vi "exchangeFormat.vi"(8 "error in TCP":errorcluster, 9 "input Controls":cluster{"name":string, "type desc":i16[]}[](array[cluster]), 10 "input Indicators":cluster{"name":string, "type desc":i16[]}[](array[cluster]), 11 "connection ID in":refnum<k5>) -> (0 "error out TCP":errorcluster, 1 "output Controls":cluster{"name":string, "type desc":i16[]}[](array[cluster]), 2 "output Indicators":cluster{"name":string, "type desc":i16[]}[](array[cluster]), 3 "connection ID out":refnum<k5>)   [LabVIEW 2010]
panel:
  out "controls":string
  out "indicators":string
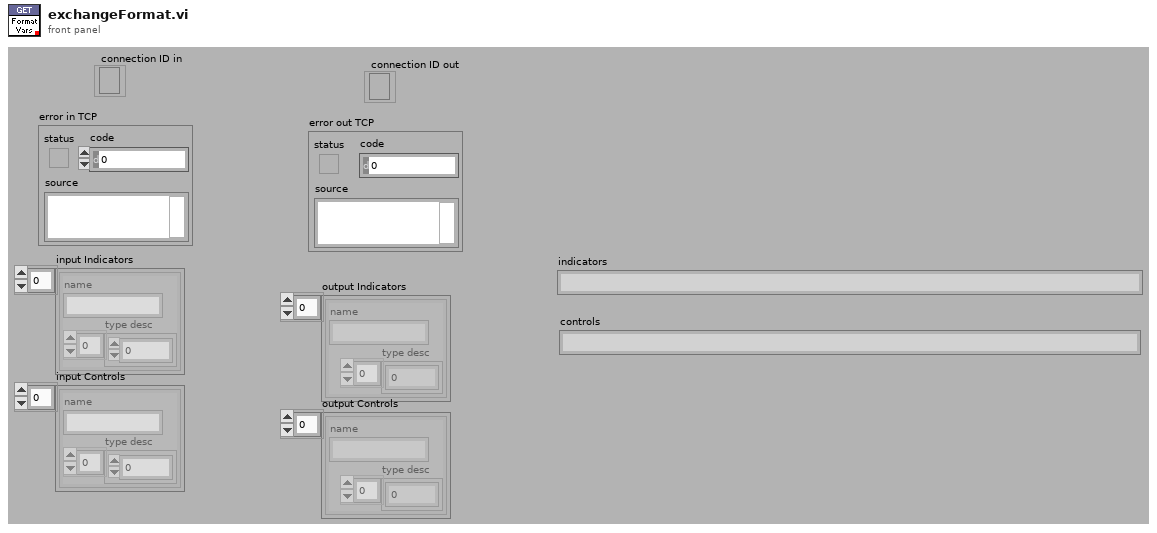
[diagram p1: front panel]
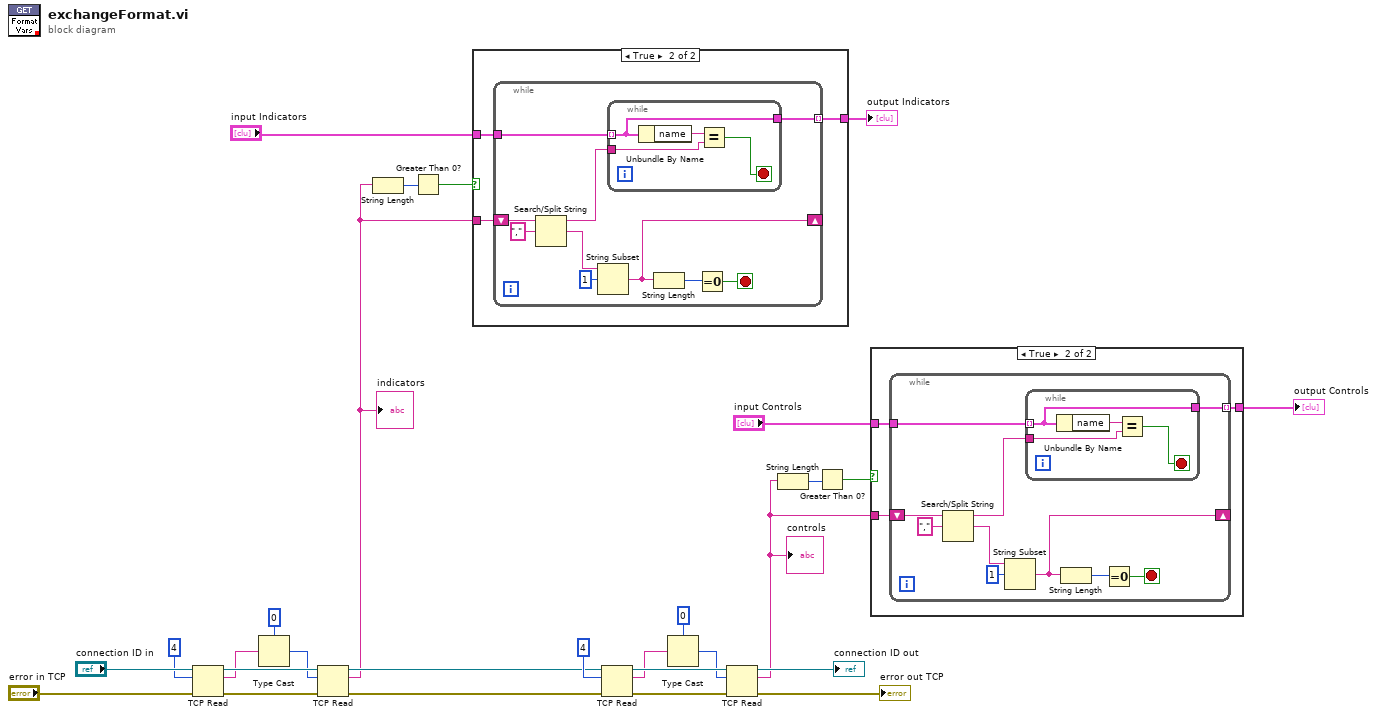
[diagram p0: block diagram]
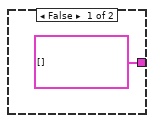
[diagram p2: hidden frame]
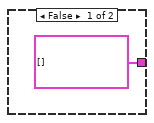
[diagram p3: hidden frame]
diagram:
  n1 = TCP Read(connection ID="connection ID in", bytes to read=4, error in (no error)="error in TCP") -> (connection ID out=w25:refnum<k5>, data out=w23:string, error out=w24:errorcluster)  [unwired: 1 in, 1 out]
  n2 = Type Cast(type=0, x=w23) -> (*(type *) &x=w21:i32)
  n3 = TCP Read(connection ID=w25, bytes to read=w21, error in (no error)=w24) -> (connection ID out=w14:refnum<k5>, data out=w6:string, error out=w13:errorcluster)  [unwired: 2 out]
  "indicators" <- w6
  n4 = String Length(string=w6) -> (length=w5:i32)
  n5 = Greater Than 0?(x=w5) -> (x > 0?=w4:bool)
  n6 = case shown="True" w4 {
    tunnel: w6 -> [_ w32]
    tunnel: [cluster{"name":string, "type desc":i16[]}[] [] w31] -> w10
    tunnel: "input Indicators" -> [_ w30]
    frame False {
    }
    frame True {
      n7 = while {
        shift-right: [w36] -> _
        shift-left: w32 -> [w41]
        tunnel: [w35] -> w31 mode=indexing
        tunnel: w30 -> [w34]
        stop <- w39 stop-if-true
        n8 = Search/Split String(string=w41, search string/char (-)=",") -> (substring before match=w33:string, match + rest of string=w38:string)  [unwired: 2 out]
        n9 = String Subset(string=w38, offset (0)=1) -> (substring=w36:string)  [unwired: 1 out]
        n10 = while {
          tunnel: w34 -> [w43] mode=indexing
          tunnel: w33 -> [w45]
          tunnel: [w43] -> w35
          stop <- w44 stop-if-true
          n11 = Unbundle By Name(w43) -> ("name"=w46:string)
          n12 = Equal?(x=w46, y=w45) -> (x = y?=w44:bool)
        }
        n13 = String Length(string=w36) -> (length=w40:i32)
        n14 = Equal To 0?(x=w40) -> (x = 0?=w39:bool)
      }
    }
  }
  "output Indicators" <- w10
  n15 = TCP Read(connection ID=w14, bytes to read=4, error in (no error)=w13) -> (connection ID out=w19:refnum<k5>, data out=w17:string, error out=w18:errorcluster)  [unwired: 1 in, 1 out]
  n16 = Type Cast(type=0, x=w17) -> (*(type *) &x=w15:i32)
  n17 = TCP Read(connection ID=w19, bytes to read=w15, error in (no error)=w18) -> (connection ID out=→"connection ID out":refnum<k5>, data out=w3:string, error out=→"error out TCP":errorcluster)  [unwired: 2 out]
  "controls" <- w3
  n18 = String Length(string=w3) -> (length=w1:i32)
  n19 = Greater Than 0?(x=w1) -> (x > 0?=w2:bool)
  n20 = case shown="True" w2 {
    tunnel: w3 -> [_ w50]
    tunnel: "input Controls" -> [_ w49]
    tunnel: [cluster{"name":string, "type desc":i16[]}[] [] w48] -> w7
    frame False {
    }
    frame True {
      n21 = while {
        shift-right: [w54] -> _
        shift-left: w50 -> [w59]
        tunnel: w49 -> [w53]
        tunnel: [w52] -> w48 mode=indexing
        stop <- w57 stop-if-true
        n22 = Search/Split String(string=w59, search string/char (-)=",") -> (substring before match=w51:string, match + rest of string=w56:string)  [unwired: 2 out]
        n23 = String Subset(string=w56, offset (0)=1) -> (substring=w54:string)  [unwired: 1 out]
        n24 = while {
          tunnel: w53 -> [w61] mode=indexing
          tunnel: w51 -> [w63]
          tunnel: [w61] -> w52
          stop <- w62 stop-if-true
          n25 = Unbundle By Name(w61) -> ("name"=w64:string)
          n26 = Equal?(x=w64, y=w63) -> (x = y?=w62:bool)
        }
        n27 = String Length(string=w54) -> (length=w58:i32)
        n28 = Equal To 0?(x=w58) -> (x = 0?=w57:bool)
      }
    }
  }
  "output Controls" <- w7
